vi "GetExternalProcesses.vi"(8 "Error In":errorcluster) -> (0 "Error Out":errorcluster, 2 "ExternalProcesses":T1[](array[typedef]))   [LabVIEW 2011]
uses:
  paramsExternalProcesses.ctl
  <vilib>/Utility/config.llb/Read Key (Path).vi
  <vilib>/Utility/config.llb/Read Key (Double).vi
  <vilib>/Utility/config.llb/Read Key (U32).vi
  <vilib>/Utility/config.llb/NI_LVConfig.lvlib
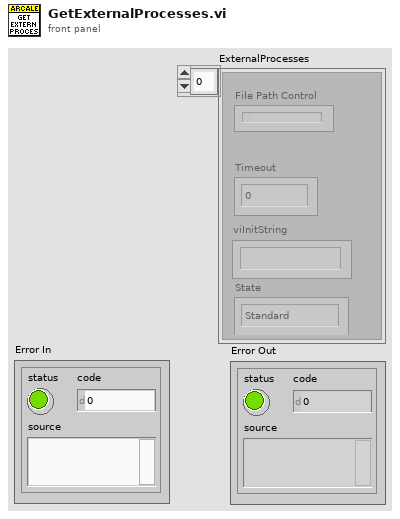
[diagram p1: front panel]
types:
  T1 = typedef "paramsExternalProcesses.ctl" = cluster{"File Path Control":path, "Timeout":dbl, "viInitString":string, "State":enum32{"Invalid", "Standard", "Closed", "Hidden", "Minimized", "Maximized"}}
  T2 = enum32{"Invalid", "Standard", "Closed", "Hidden", "Minimized", "Maximized"}
  T3 = typedef "ApplicationPaths.ctl" = cluster{"Data Path":path, "Log Path":path, "Tmp Path":path}
  T4 = typedef "NI_LVConfig.lvlib/Config Data RefNum.ctl" = refnum<k1>
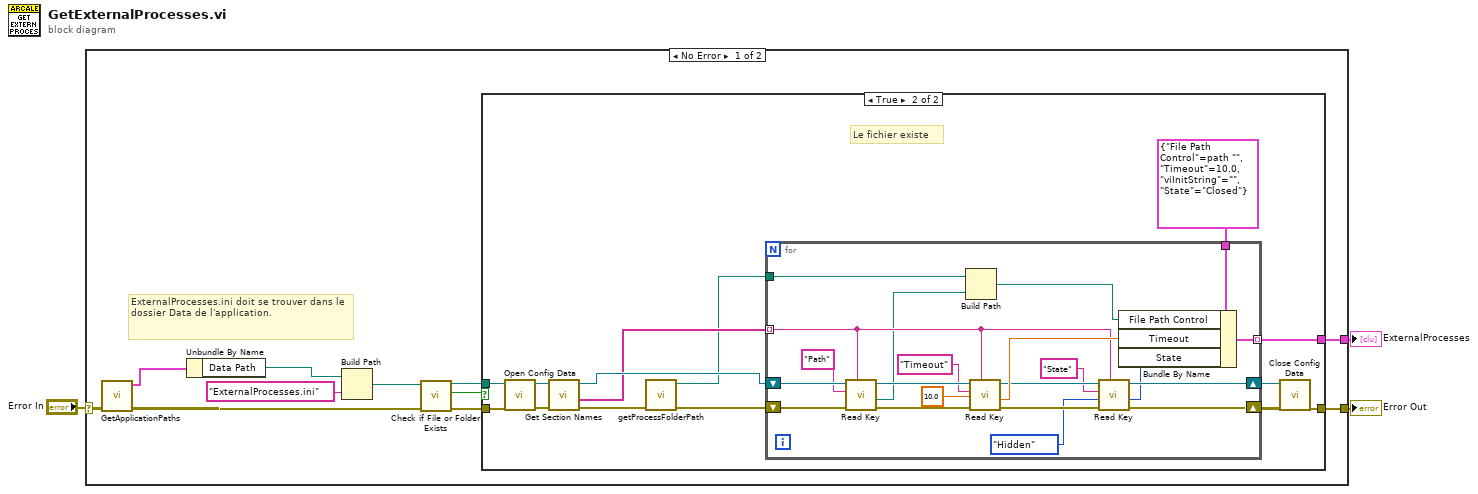
[diagram p0: block diagram]
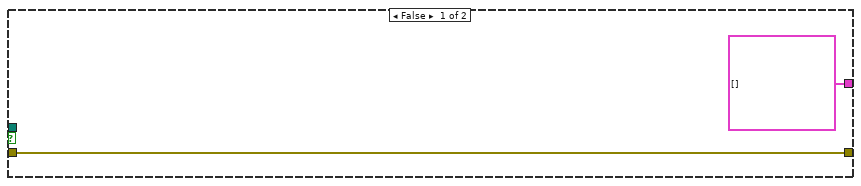
[diagram p2: hidden frame]
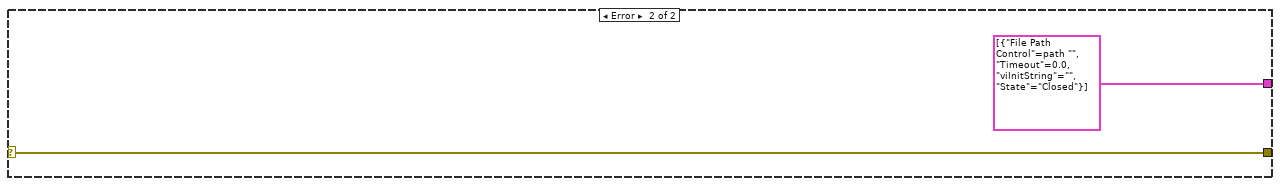
[diagram p3: hidden frame]
diagram:
  n1 = case shown="No Error" "Error In" {
    selector: "Error In" -> [w11 w53]
    tunnel: [w13 w53] -> w3
    tunnel: [w14 T1[] [{"File Path Control"=path "", "Timeout"=0.0, "viInitString"="", "State"=enum."Closed"}]] -> w1
    frame No Error {
      # "ExternalProcesses.ini doit se trouver dans le dossier Data de l'application."
      n2 = call "GetApplicationPaths.vi"("error in (no error)"=w11) -> ("error out"=w8:errorcluster, "ApplicationPath"=w10:T3)  [unwired: 9 in]
      n3 = Unbundle By Name(w10) -> ("Data Path"=w9:path)
      n4 = Build Path(base path=w9, name or relative path="ExternalProcesses.ini") -> (appended path=w4:path)
      n5 = call <vilib>:"Check if File or Folder Exists.vi"("error in (no error)"=w8, "path"=w4) -> ("error out"=w7:errorcluster, "file or folder exists?"=w5:bool, "dup path"=w6:path)  [unwired: 7 in]
      n6 = case shown="True" w5 {
        tunnel: [T1[] [] w30] -> w14
        tunnel: [w16 w29] -> w13
        tunnel: w7 -> [w16 w18]
        tunnel: w6 -> [_ w17]
        frame False {
        }
        frame True {
          # "Le fichier existe"
          n7 = call <vilib>:"Open Config Data.vi"("error in (no error)"=w18, "configuration file path"=w17) -> ("error out"=w26:errorcluster, "refnum"=w27:T4)  [unwired: 7 in, 1 out]
          n8 = call <vilib>:"Get Section Names.vi"("error in (no error)"=w26, "refnum"=w27) -> ("error out"=w20:errorcluster, "section names"=w24:string[], "refnum out"=w25:T4)  [unwired: 7 in]
          n9 = call "getProcessFolderPath.vi"("error in (no error)"=w20) -> ("error out"=w19:errorcluster, "Process Folder"=w21:path)  [unwired: 9 in]
          n10 = for {
            shift-right: [w38] -> w22
            shift-left: w19 -> [w51]
            tunnel: w24 -> [w34] mode=indexing
            shift-right: [w39] -> w23
            shift-left: w25 -> [w50]
            tunnel: [w43] -> w30 mode=indexing
            tunnel: T1 {"File Path Control"=path "", "Timeout"=10.0, "viInitString"="", "State"=enum."Closed"} -> [w42]
            tunnel: w21 -> [w31]
            n11 = call-poly <vilib>:"Read Key.vi"("section"=w34, "error in (no error)"=w51, "key"="Path", "refnum"=w50) -> ("error out"=w49:errorcluster, "value"=w33:path, "refnum out"=w47:T4)  [unwired: 4 in, 1 out]
            n12 = Build Path(base path=w31, name or relative path=w33) -> (appended path=w32:path)
            n13 = call-poly <vilib>:"Read Key.vi"("section"=w34, "error in (no error)"=w49, "default value"=10.0, "key"="Timeout", "refnum"=w47) -> ("error out"=w41:errorcluster, "value"=w45:dbl, "refnum out"=w40:T4)  [unwired: 3 in, 1 out]
            n14 = call-poly <vilib>:"Read Key.vi"("section"=w34, "error in (no error)"=w41, "default value"=T2."Hidden" ("State"), "key"="State", "refnum"=w40) -> ("error out"=w38:errorcluster, "value"=w35:u32, "refnum out"=w39:T4)  [unwired: 3 in, 1 out]
            n15 = Bundle By Name(cluster=w42, "File Path Control"=w32, "Timeout"=w45, "State"=w35) -> (w43:T1)
          }
          n16 = call <vilib>:"Close Config Data.vi"("error in (no error)"=w22, "refnum"=w23) -> ("error out"=w29:errorcluster)  [unwired: 8 in, 1 out]
        }
      }
    }
    frame Error {
    }
  }
  "Error Out" <- w3
  "ExternalProcesses" <- w1
